vi "CT_ScaleMagCurrent.vi"(8 "Offset Array":dbl[](array[numeric])=[-740.0, -389.0, -360.0, -410.0], 9 "Slope Array":dbl[](array[numeric])=[909.6, 232.5, 306.0, 333.8], 10 "DAQ Meas":waveform(dbl)[](graph)=[{"t0"=timestamp(3354657826.5396585 s since 1904-01-01), "dt"=0.0033333, "Y"=array[1000 elements], "attributes"=variant("NI_ChannelName"=variant(string "Current_CoilC"), "NI_UnitDescription"=variant(string "Volts"))}, {"t0"=timestamp(3354657826.5396724 s since 1904-01-01), "dt"=0.0033333, "Y"=array[1000 elements], "attributes"=variant("NI_ChannelName"=variant(string "Current_CoilB"), "NI_UnitDescription"=variant(string "Volts"))}, {"t0"=timestamp(3354657826.5396867 s since 1904-01-01), "dt"=0.0033333, "Y"=array[1000 elements], "attributes"=variant("NI_ChannelName"=variant(string "Current_CoilA"), "NI_UnitDescription"=variant(string "Volts"))}]) -> (2 "Converted to Amps":waveform(dbl)[](graph)=[{"t0"=timestamp(3354657826.5396585 s since 1904-01-01), "dt"=0.0033333, "Y"=array[1000 elements], "attributes"=variant("NI_ChannelName"=variant(string "Current_CoilC"), "NI_UnitDescription"=variant(string "Volts"))}, {"t0"=timestamp(3354657826.5396724 s since 1904-01-01), "dt"=0.0033333, "Y"=array[1000 elements], "attributes"=variant("NI_ChannelName"=variant(string "Current_CoilB"), "NI_UnitDescription"=variant(string "Volts"))}, {"t0"=timestamp(3354657826.5396867 s since 1904-01-01), "dt"=0.0033333, "Y"=array[1000 elements], "attributes"=variant("NI_ChannelName"=variant(string "Current_CoilA"), "NI_UnitDescription"=variant(string "Volts"))}])   [LabVIEW 2016]
panel:
  out "Array":string[](array[string])
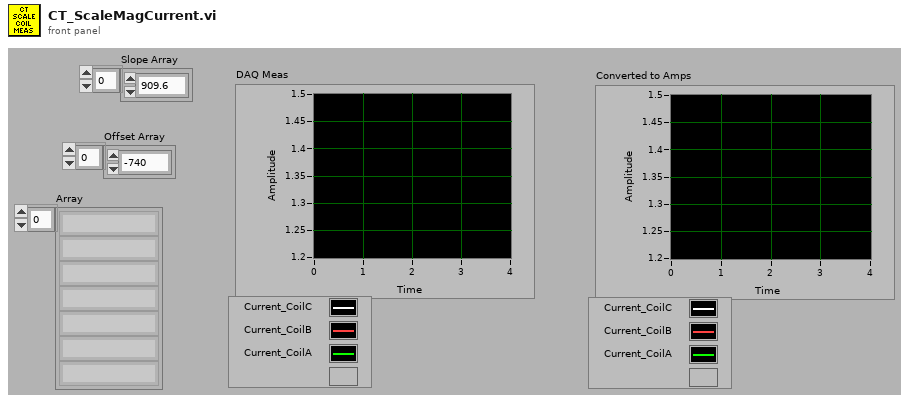
[diagram p1: front panel]
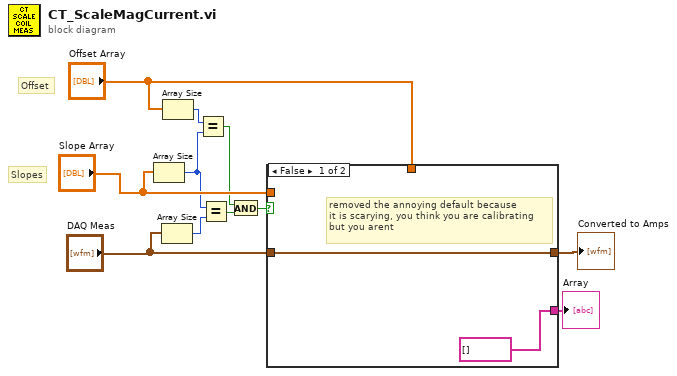
[diagram p0: block diagram]
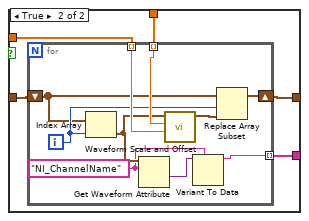
[diagram p2: hidden frame]
diagram:
  # "Offset"
  # "Slopes"
  n1 = Array Size(array="Slope Array") -> (size(s)=w6:i32)
  n2 = Array Size(array="DAQ Meas") -> (size(s)=w5:i32)
  n3 = Array Size(array="Offset Array") -> (size(s)=w7:i32)
  n4 = Equal?(x=w7, y=w6) -> (x = y?=w4:bool)
  n5 = Equal?(x=w6, y=w5) -> (x = y?=w3:bool)
  n6 = And(x=w4, y=w3) -> (x .and. y?=w2:bool)
  n7 = case shown="False" w2 {
    tunnel: [w12 w18] -> w11
    tunnel: "DAQ Meas" -> [w12 w17]
    tunnel: "Slope Array" -> [_ w16]
    tunnel: "Offset Array" -> [_ w15]
    tunnel: [string[] [] w14] -> w1
    frame False {
      # "removed the annoying default because\nit is scarying, you think you are calibrating\nbut you arent"
    }
    frame True {
      n8 = for {
        tunnel: w16 -> [w28] mode=indexing
        tunnel: w15 -> [w27] mode=indexing
        shift-right: [w24] -> w18
        shift-left: w17 -> [w23]
        tunnel: [w19] -> w14 mode=indexing
        i -> [w26]
        w20 = "NI_ChannelName" ("name")
        n9 = Index Array(array=w23, index=w26) -> (element=w22:waveform(dbl))
        n10 = Get Waveform Attribute(6:w20, 7:w22) -> (1:w21:variant)  [unwired: 2 in, 3 out]
        n11 = call <vilib>:"Waveform Scale and Offset.vi"("scale"=w28, "offset"=w27, "waveform in"=w22) -> ("waveform out"=w25:waveform(dbl))  [unwired: 7 in, 1 out]
        n12 = Variant To Data(type=w20, Variant=w21) -> (data=w19:string)  [unwired: 1 in, 1 out]
        n13 = Replace Array Subset(array=w23, new element=w25, index=w26) -> (w24:waveform(dbl)[])
      }
    }
  }
  "Converted to Amps" <- w11
  "Array" <- w1
